vi "UDP Data Link - Configuration Utilities - Initialize Device Properties.vi"(8 "error in (no error)":errorcluster, 11 "Device Item Ref in":T1 format="%.0x") -> (0 "error out":errorcluster, 3 "Item Ref out":T1 format="%.0x")   [LabVIEW 2012, in "UDP Data Link System Explorer.lvlib"]
doc: "Initialize the UDP Data Link custom device properties."
uses:
  UDP Data Link System Explorer.lvlib
  <vilib>/NI Veristand/Custom Device API/Custom Device Item Ref.ctl
  Shared/UDP Data Link Global.vi
  <vilib>/NI Veristand/Custom Device API/Set Item Property (Boolean).vi
  <vilib>/NI Veristand/Custom Device API/Set Item Property (Path).vi
  <vilib>/NI Veristand/Custom Device API/Set Item Property (I32).vi
  <vilib>/NI Veristand/Custom Device API/Set Item Property (String).vi
  <vilib>/NI Veristand/Custom Device API/Set Item Property (U16).vi
  <vilib>/NI Veristand/Custom Device API/Custom Device API.lvlib
  Shared/UDP Data Link Shared.lvlib
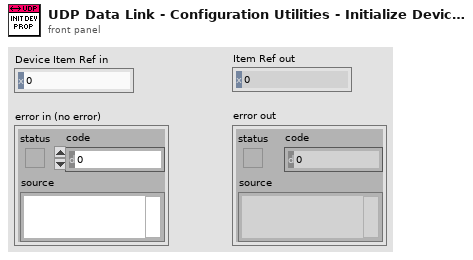
[diagram p1: front panel]
types:
  T1 = typedef "Custom Device API.lvlib/Custom Device Item Ref.ctl" = u64
  T2 = enum8{"Enabled", "Disabled", "Disabled and Grayed Out"}
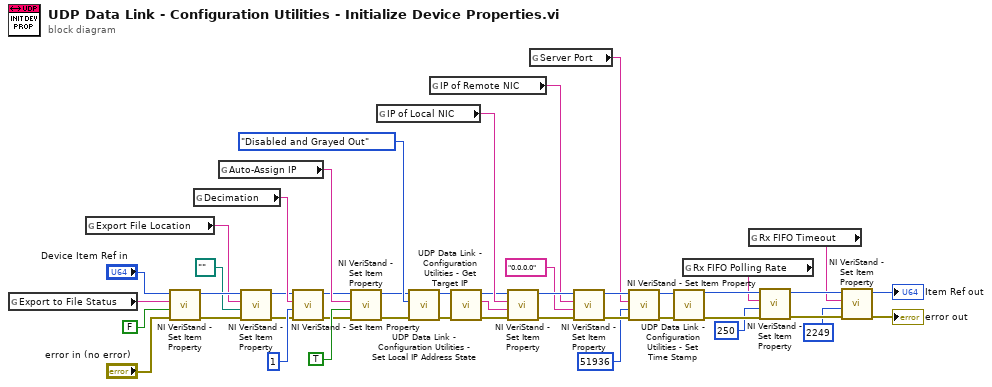
[diagram p0: block diagram]
diagram:
  n1 = global read "UDP Data Link Global.vi" "Export to File Status"() -> (w20:string)
  n2 = global read "UDP Data Link Global.vi" "Export File Location"() -> (w13:string)
  n3 = call-poly <vilib>:"NI VeriStand - Set Item Property.vi"("error in (no error)"="error in (no error)", "Value"=FALSE, "Property Name"=w20, "Item Ref in"="Device Item Ref in") -> ("error out"=w16:errorcluster, "Item Ref out"=w18:T1)  [unwired: 5 in, 1 out]
  n4 = global read "UDP Data Link Global.vi" "Decimation"() -> (w22:string)
  n5 = global read "UDP Data Link Global.vi" "Auto-Assign IP"() -> (w27:string)
  n6 = call-poly <vilib>:"NI VeriStand - Set Item Property.vi"("error in (no error)"=w16, "Value"=path "", "Property Name"=w13, "Item Ref in"=w18) -> ("error out"=w14:errorcluster, "Item Ref out"=w17:T1)  [unwired: 5 in, 1 out]
  n7 = call-poly <vilib>:"NI VeriStand - Set Item Property.vi"("error in (no error)"=w14, "Value"=1, "Property Name"=w22, "Item Ref in"=w17) -> ("error out"=w23:errorcluster, "Item Ref out"=w24:T1)  [unwired: 5 in, 1 out]
  n8 = call-poly <vilib>:"NI VeriStand - Set Item Property.vi"("error in (no error)"=w23, "Value"=TRUE, "Property Name"=w27, "Item Ref in"=w24) -> ("error out"=w28:errorcluster, "Item Ref out"=w26:T1)  [unwired: 5 in, 1 out]
  n9 = global read "UDP Data Link Global.vi" "IP of Local NIC"() -> (w37:string)
  n10 = call "UDP Data Link - Configuration Utilities - Set Local IP Address State.vi"("error in (no error)"=w28, "State"=T2."Disabled and Grayed Out", "Item Ref in"=w26) -> ("error out"=w31:errorcluster, "Item Ref out"=w30:T1)  [unwired: 7 in]
  n11 = global read "UDP Data Link Global.vi" "IP of Remote NIC"() -> (w39:string)
  n12 = call "UDP Data Link - Configuration Utilities - Get Target IP.vi"("error in"=w31, "Item Ref in"=w30) -> ("error out"=w33:errorcluster, "IPAddress"=w32:string, "Item Ref out"=w34:T1)  [unwired: 7 in]
  n13 = call-poly <vilib>:"NI VeriStand - Set Item Property.vi"("error in (no error)"=w33, "Value"=w32, "Property Name"=w37, "Item Ref in"=w34) -> ("error out"=w40:errorcluster, "Item Ref out"=w41:T1)  [unwired: 5 in, 1 out]
  n14 = global read "UDP Data Link Global.vi" "Server Port"() -> (w43:string)
  n15 = call-poly <vilib>:"NI VeriStand - Set Item Property.vi"("error in (no error)"=w40, "Value"="0.0.0.0", "Property Name"=w39, "Item Ref in"=w41) -> ("error out"=w44:errorcluster, "Item Ref out"=w45:T1)  [unwired: 5 in, 1 out]
  n16 = call-poly <vilib>:"NI VeriStand - Set Item Property.vi"("error in (no error)"=w44, "Value"=u16 51936, "Property Name"=w43, "Item Ref in"=w45) -> ("error out"=w36:errorcluster, "Item Ref out"=w35:T1)  [unwired: 5 in, 1 out]
  n17 = call "UDP Data Link - Configuration Utilities - Set Time Stamp.vi"("error in (no error)"=w36, "Device Item Ref in"=w35) -> ("error out"=w10:errorcluster, "Device Item Ref out"=w9:T1)  [unwired: 7 in, 1 out]
  n18 = global read "UDP Data Link Global.vi" "Rx FIFO Polling Rate"() -> (w8:string)
  n19 = global read "UDP Data Link Global.vi" "Rx FIFO Timeout"() -> (w4:string)
  n20 = call-poly <vilib>:"NI VeriStand - Set Item Property.vi"("error in (no error)"=w10, "Value"=u16 250, "Property Name"=w8, "Item Ref in"=w9) -> ("error out"=w6:errorcluster, "Item Ref out"=w5:T1)  [unwired: 5 in, 1 out]
  n21 = call-poly <vilib>:"NI VeriStand - Set Item Property.vi"("error in (no error)"=w6, "Value"=u16 2249, "Property Name"=w4, "Item Ref in"=w5) -> ("error out"=→"error out":errorcluster, "Item Ref out"=→"Item Ref out":T1)  [unwired: 5 in, 1 out]
